vi "Stop Core.vi"(10 "final error code":i32, 11 "Filter Config Display in":refnum<class "Filter Config Display.lvclass">) -> (3 "Filter Config Display out":refnum<class "Filter Config Display.lvclass">)   [LabVIEW 2016, in "Assert API Components.lvlib" / "Assert Display.lvlib" / "Filter Config Display.lvlib" / "Filter Config Display.lvclass"]
doc: "(<B>Filename</B>: Actor Framework.lvlib:Actor.lvclass:Stop Core.vi)\n\nDefines what the actor does before it stops. Use the <B>final error code</B> input to determine whether the actor shut down in response to an error.\n\nBy default, this method does nothing. A descendant class may override it to define behavior, such as shutting down any processes the actor initiated in its override of the Actor Core method."
uses:
  Filter Config Display.lvclass
  Filter Config Display.lvclass/Filter Config Display.ctl
  Base UI Component/Base UI Component/Base UI Component.lvclass
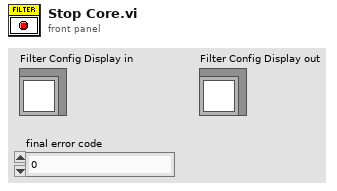
[diagram p1: front panel]
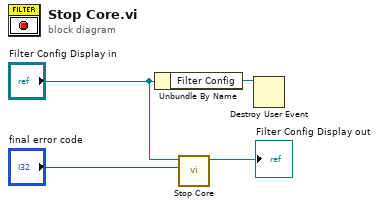
[diagram p0: block diagram]
diagram:
  n1 = Unbundle By Name("Filter Config Display in") -> ("Filter Config"=w1:refnum<user-event>)
  n2 = call-parent "Stop Core.vi"("final error code"="final error code", "Base UI Component in"="Filter Config Display in") -> ("Base UI Component out"=→"Filter Config Display out":refnum<class "Filter Config Display.lvclass">)  [unwired: 9 in]
  n3 = Destroy User Event(user event=w1) -> ()  [unwired: 1 in, 1 out]
